vi "Write timeout.vi"(10 "timeout":i32=1000, 11 "Properties.Suite in":refnum<class "Properties.Suite.lvclass">) -> (3 "Properties.Suite out":refnum<class "Properties.Suite.lvclass">)   [LabVIEW 2020, in "Caraya.lvlib" / "Properties.Suite.lvclass"]
uses:
  Properties.Suite.lvclass
  Properties.Suite.lvclass/Properties.Suite.ctl
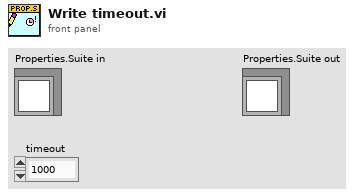
[diagram p1: front panel]
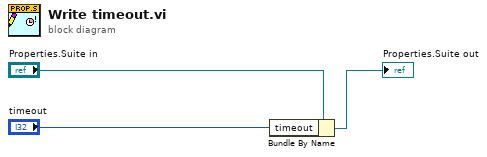
[diagram p0: block diagram]
diagram:
  n1 = Bundle By Name(cluster="Properties.Suite in", "timeout"="timeout") -> (→"Properties.Suite out":refnum<class "Properties.Suite.lvclass">)
